vi "Check Contains.vi"(10 "Segment B":i32[](array[numeric]), 11 "Segment A":i32[](array[numeric])) -> (3 "A Contains B?":bool)   [LabVIEW 2020]
panel:
  out "Extra In B":i32
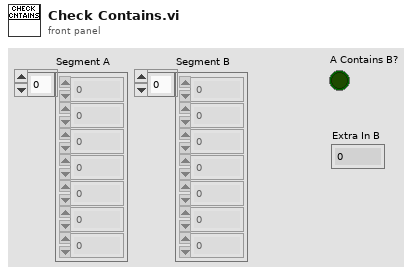
[diagram p1: front panel]
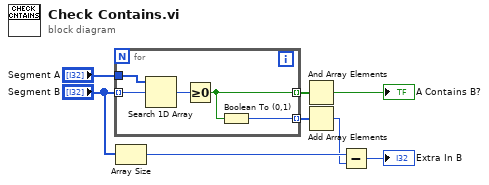
[diagram p0: block diagram]
diagram:
  n1 = for {
    tunnel: "Segment B" -> [w13] mode=indexing
    tunnel: [w10] -> w7 mode=indexing
    tunnel: "Segment A" -> [w11]
    tunnel: [w9] -> w5 mode=indexing
    n2 = Search 1D Array(1D array=w11, element=w13) -> (index of element=w12:i32)  [unwired: 1 in]
    n3 = Greater Or Equal To 0?(x=w12) -> (x >= 0?=w10:bool)
    n4 = Boolean To (0,1)(Boolean=w10) -> (0, 1=w9:i16)
  }
  n5 = Array Size(array="Segment B") -> (size(s)=w3:i32)
  n6 = And Array Elements(Boolean array=w7) -> (logical AND=→"A Contains B?":bool)
  n7 = Add Array Elements(numeric array=w5) -> (sum=w2:i16)
  n8 = Subtract(x=w3, y=w2) -> (x-y=→"Extra In B":i32)
